vi "Read Time.vi"(8 "error in (no error)":errorcluster, 11 "ControlDropMsg In":refnum<class "ControlDropMsg.lvclass">) -> (0 "error out":errorcluster, 2 "Time":u32, 3 "ControlDropMsg Out":refnum<class "ControlDropMsg.lvclass">)   [LabVIEW 2017, in "ActorEvents.lvlib" / "ControlDropMsg.lvclass"]
uses:
  ControlDropMsg.lvclass
  ControlDropMsg.lvclass/ControlDropMsg.ctl
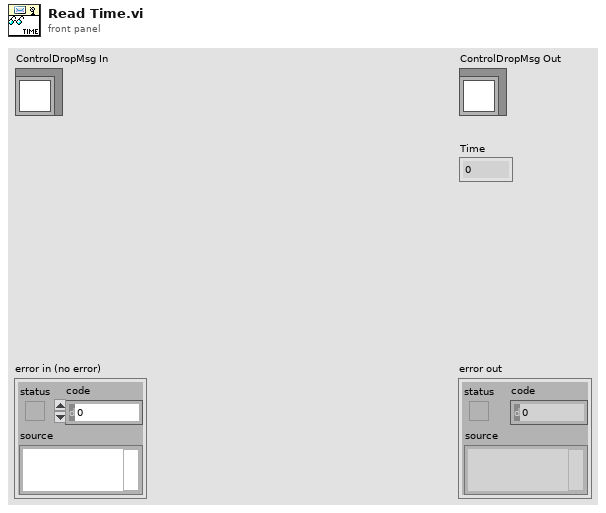
[diagram p1: front panel]
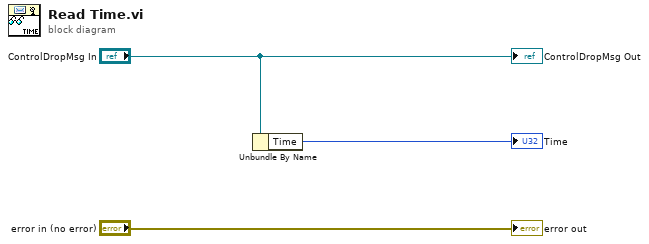
[diagram p0: block diagram]
diagram:
  n1 = Unbundle By Name("ControlDropMsg In") -> ("Time"=→"Time":u32)
  "error out" <- "error in (no error)"
  "ControlDropMsg Out" <- "ControlDropMsg In"
